vi "FTW-Container-Support-JSON-ParseCompositeType.vi"(0 "JSON String":string, 5 "Expected Type":T1=enum."Array", 11 "error in":errorcluster) -> (4 "Elements":T2[](array[typedef]), 15 "error out":errorcluster)   [LabVIEW 2014, in "FTW-Container.lvclass"]
uses:
  FTW-Container.lvclass
  FTW-Container-Support-JSON-ElementToProcess.ctl
  JSON/FTW-JSON-Datatype.ctl
  JSON/FTW-JSON-CompositeType.ctl
  Regex/FTW-Regex.vi
  Error/FTW-ERR-ThrowError.vi
  JSON/FTW-JSON-RegexHeader.vi
panel:
  # "Inputs"
  # "Outputs"
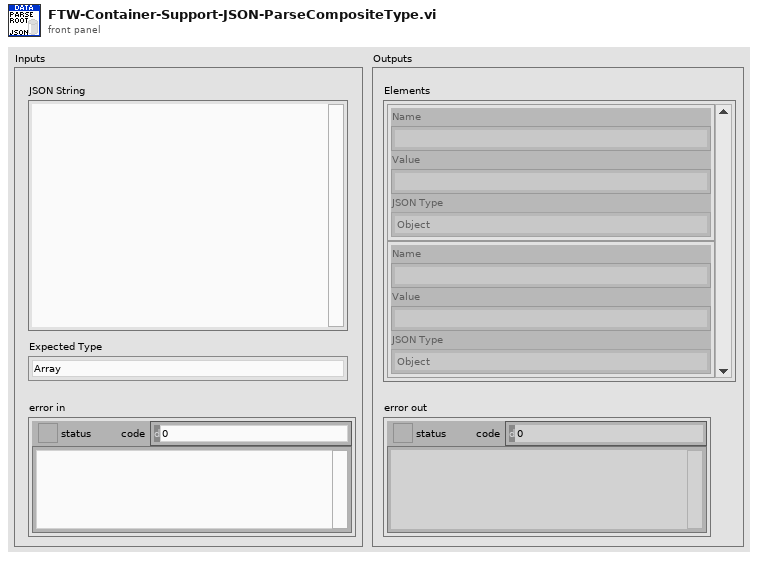
[diagram p1: front panel]
types:
  T1 = typedef "FTW-JSON-CompositeType.ctl" = enum16{"Object", "Array"}
  T2 = typedef "FTW-Container.lvclass/FTW-Container-Support-JSON-ElementToProcess.ctl" = cluster{"Name":string, "Value":string, "JSON Type":T3}
  T3 = typedef "FTW-JSON-Datatype.ctl" = enum16{"Object", "Array", "String", "Number", "Boolean", "NULL", "<Refnum>", "<Enum>", "<Unknown>"}
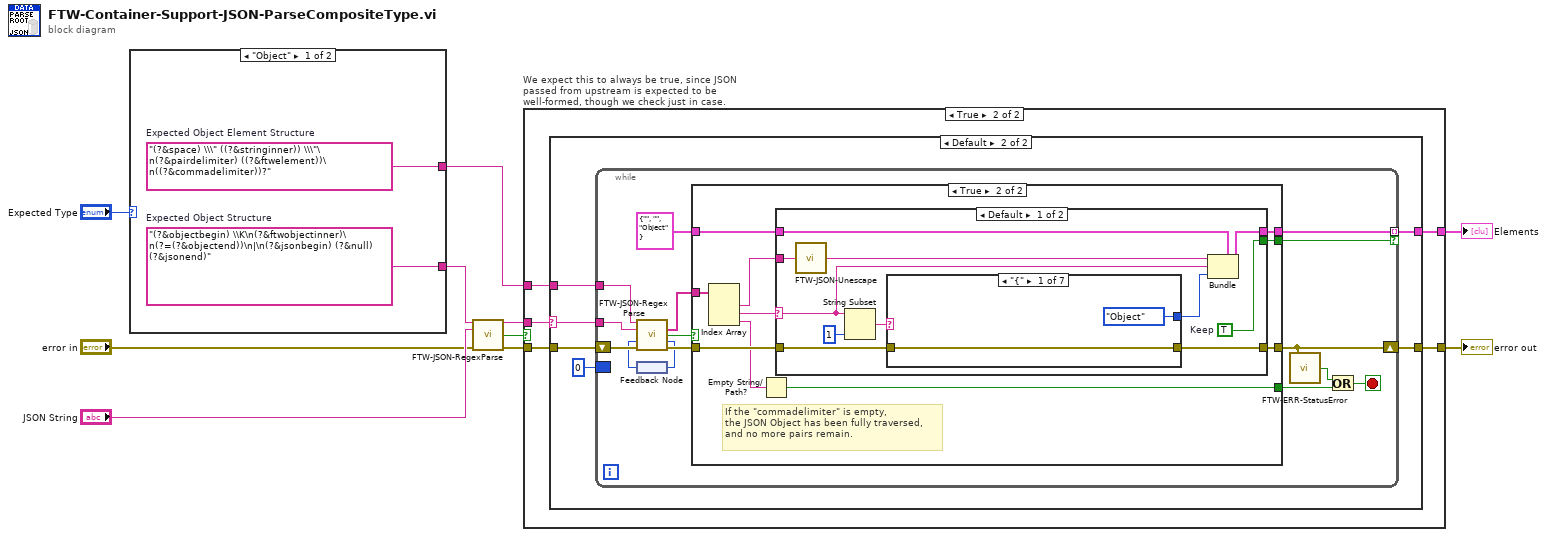
[diagram p0: block diagram]
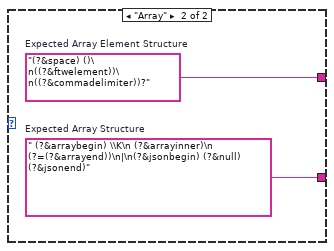
[diagram p2: hidden frame]
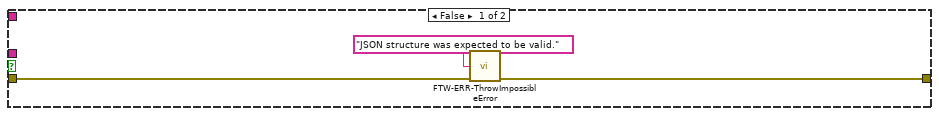
[diagram p3: hidden frame]
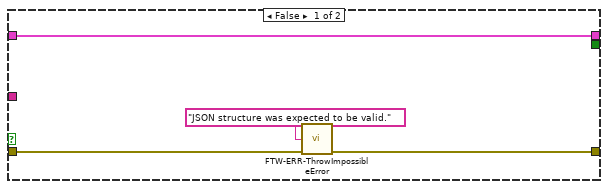
[diagram p5: hidden frame]
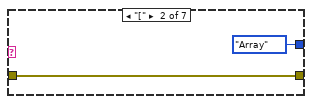
[diagram p6: hidden frame]
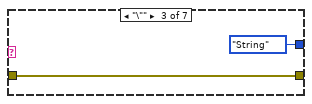
[diagram p7: hidden frame]
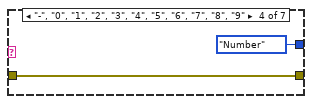
[diagram p8: hidden frame]
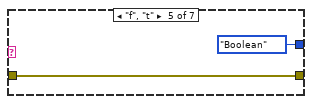
[diagram p9: hidden frame]
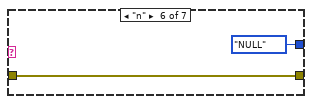
[diagram p10: hidden frame]
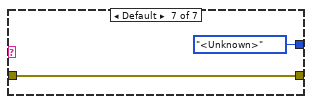
[diagram p11: hidden frame]
diagram:
  n1 = case shown="\"Object\"" "Expected Type" {
    tunnel: [w12 w14] -> w8
    tunnel: [w11 w13] -> w6
    frame "Object" {
      w12 = "(?&space) \\\" ((?&stringinner)) \\\"\n(?&pairdelimiter) ((?&ftwelement))\n((?&commadelimiter))?"  # Expected Object Element Structure
      w11 = "(?&objectbegin) \\K\n(?&ftwobjectinner)\n(?=(?&objectend))\n|\n(?&jsonbegin) (?&null) (?&jsonend)"  # Expected Object Structure
    }
    frame "Array" {
      w14 = "(?&space) ()\n((?&ftwelement))\n((?&commadelimiter))?"  # Expected Array Element Structure
      w13 = " (?&arraybegin) \\K\n (?&arrayinner)\n (?=(?&arrayend))\n|\n(?&jsonbegin) (?&null) (?&jsonend)"  # Expected Array Structure
    }
  }
  n2 = call "FTW-JSON-RegexParse.vi"("Regular Expression using JSON subroutines"=w6, "Input String"="JSON String", "error in"="error in") -> ("Match"=w5:string, "Found Match?"=w2:bool, "error out"=w4:errorcluster)  [unwired: 8 in, 2 out]
  n3 = case "We expect this to always be true, since JSON passed from upstream is expected to be well-formed, though we check just in case." shown="True" w2 {
    tunnel: [w15 w22] -> w9
    tunnel: w8 -> [_ w21]
    tunnel: w5 -> [_ w20]
    tunnel: w4 -> [w16 w19]
    tunnel: [_ w18] -> w3
    frame False {
      n4 = call "FTW-ERR-ThrowImpossibleError.vi"("Reason this error should never happen"="JSON structure was expected to be valid.", "error in"=w16) -> ("error out"=w15:errorcluster)  [unwired: 13 in]
    }
    frame True {
      n5 = case shown="Default" w20 {
        selector: w20 -> [_ w27]
        tunnel: [w23 w29] -> w22
        tunnel: w19 -> [w23 w25]
        tunnel: w21 -> [_ w28]
        tunnel: [_ w24] -> w18
        frame "", "null" {
          # "<< Case Insensitive Match turned on -- silently ignore null objects for now."
        }
        frame Default {
          n6 = while {
            tunnel: w27 -> [w43]
            shift-right: [w37] -> w29
            shift-left: w25 -> [w44]
            border: 0 -> [_]
            tunnel: w28 -> [w33]
            tunnel: [w32] -> w24 mode=indexing if=w31
            stop <- w34 stop-if-true
            n7 = feedback #1() -> (w41:i32)
            n8 = call "FTW-JSON-RegexParse.vi"("Regular Expression using JSON subroutines"=w33, "Input String"=w43, "Starting Offset"=w41, "error in"=w44) -> ("Submatches"=w38:string[], "Found Match?"=w40:bool, "Offset after Match"=w39:i32, "error out"=w42:errorcluster)  [unwired: 7 in, 1 out]
            n9 = feedback-in #1(w39) -> ()
            n10 = case shown="True" w40 {
              tunnel: [w46 w57] -> w37
              tunnel: w42 -> [w47 w58]
              tunnel: [_ w52] -> w36
              tunnel: w38 -> [_ w56]
              tunnel: [w45 w54] -> w32
              tunnel: [_ w53] -> w31
              tunnel: T2 {"Name"="", "Value"="", "JSON Type"=enum."Object"} -> [w45 w51]
              frame False {
                n11 = call "FTW-ERR-ThrowImpossibleError.vi"("Reason this error should never happen"="JSON structure was expected to be valid.", "error in"=w47) -> ("error out"=w46:errorcluster)  [unwired: 13 in]
              }
              frame True {
                # "If the \"commadelimiter\" is empty,\nthe JSON Object has been fully traversed,\nand no more pairs remain."
                n12 = Index Array(array=w56) -> (element #1=w49:string, element #2=w50:string, element #3=w55:string)  [unwired: 3 in]
                n13 = Empty String/Path?(string/path=w55) -> (empty?=w52:bool)
                n14 = case shown="Default" w50 {
                  selector: w50 -> [w61 _]
                  tunnel: w58 -> [w69 w84]
                  tunnel: [w68 w84] -> w57
                  tunnel: w49 -> [w60 _]
                  tunnel: [w67 w85] -> w54
                  tunnel: [w66 _] -> w53
                  tunnel: w51 -> [w62 w85]
                  frame Default {
                    w66 = TRUE  # Keep
                    n15 = call "FTW-JSON-Unescape.vi"("Escaped UTF-8 String"=w60) -> ("Unescaped String"=w59:string)
                    n16 = String Subset(string=w61, length (rest)=1 ("length (rest)")) -> (substring=w64:string)  [unwired: 1 in]
                    n17 = case shown="\"{\"" w64 {
                      tunnel: w69 -> [w70 w72 w74 w76 w78 w80 w82]
                      tunnel: [FTW-JSON-Datatype."Object" ("JSON Type") FTW-JSON-Datatype."Array" ("JSON Type") FTW-JSON-Datatype."String" ("JSON Type") FTW-JSON-Datatype."Number" ("JSON Type") FTW-JSON-Datatype."Boolean" ("JSON Type") FTW-JSON-Datatype."NULL" ("JSON Type") FTW-JSON-Datatype."<Unknown>" ("JSON Type")] -> w63
                      tunnel: [w70 w72 w74 w76 w78 w80 w82] -> w68
                      frame "{" {
                      }
                      frame "[" {
                      }
                      frame "\"" {
                      }
                      frame "-", "0", "1", "2", "3", "4", "5", "6", "7", "8", "9" {
                      }
                      frame "f", "t" {
                      }
                      frame "n" {
                      }
                      frame Default {
                      }
                    }
                    n18 = Bundle(cluster=w62, "Name"=w59, "Value"=w61, "JSON Type"=w63) -> (w67:T2)
                  }
                  frame "null" {
                  }
                }
              }
            }
            n19 = call "FTW-ERR-StatusError.vi"("error to check"=w37) -> ("Error?"=w35:bool)
            n20 = Or(x=w35, y=w36) -> (x .or. y?=w34:bool)
          }
        }
      }
    }
  }
  "error out" <- w9
  "Elements" <- w3
